vi "testReadNotifierServerStatus_cmd.vi"(8 "error in (no error)":errorcluster) -> (0 "error out":errorcluster)   [LabVIEW 2018]
doc: "Test the readNotifierServerStatus.vi with cmd selection."
uses:
  src/TcpServer/TcpServer.lvclass
  src/TcpServer/TcpServer.lvclass/TcpServer.ctl
  src/TcpServerBase/TcpServerBase.lvclass/TcpServerBase.ctl
  src/TcpServerCmd/TcpServerCmd.lvclass
  home/pcortes/Documents/github/ts_labview_tcp_json/src/TcpServerBase/TcpServerBase.lvclass
  <vilib>/addons/_JKI Toolkits/Caraya/classes/Assert/Assert Equal Type_Variant.vi
  <vilib>/addons/_JKI Toolkits/Caraya/classes/Test/Test.lvclass
  <vilib>/addons/_JKI Toolkits/Caraya/classes/Assert/Assert.lvclass
  src/TcpServerBase/TcpServerBase.lvclass
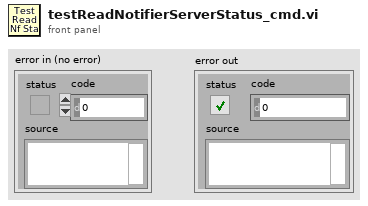
[diagram p1: front panel]
types:
  T1 = cluster{"connectionStatus":bool, "errorSource":string}
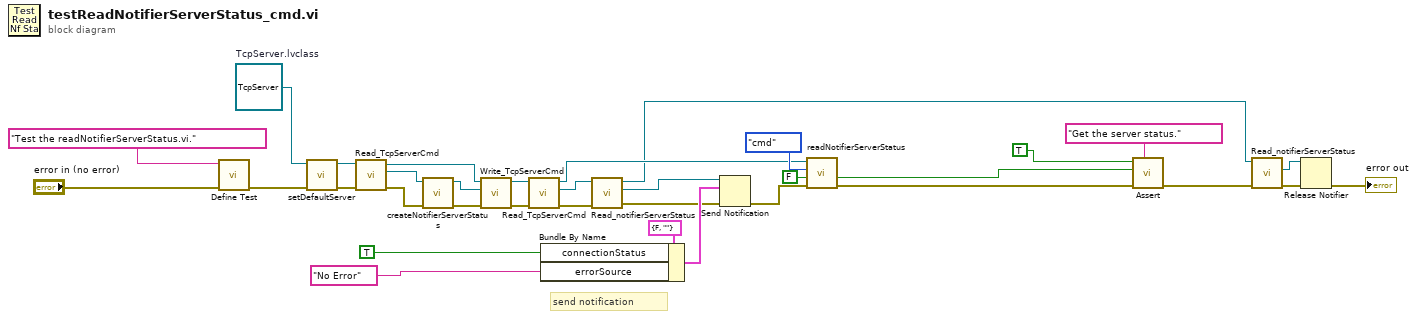
[diagram p0: block diagram]
diagram:
  w29 = refnum<class "TcpServer.lvclass"> refnum  # TcpServer.lvclass
  # "send notification"
  n1 = call <vilib>:"Define Test.vi"("error in (no error)"="error in (no error)", "Label (VI Title)"="Test the readNotifierServerStatus.vi.") -> ("error out"=w28:errorcluster)  [unwired: 9 in]
  n2 = call "setDefaultServer.vi"("error in (no error)"=w28, "TcpServer.lvclass"=w29) -> ("error out"=w27:errorcluster, "tcpServer out"=w26:refnum<class "TcpServer.lvclass">)  [unwired: 8 in]
  n3 = call "Read_TcpServerCmd.vi"("error in (no error)"=w27, "TcpServer in"=w26) -> ("error out"=w12:errorcluster, "TcpServerCmd.lvclass"=w13:refnum<class "TcpServerCmd.lvclass">, "TcpServer out"=w11:refnum<class "TcpServer.lvclass">)  [unwired: 7 in]
  n4 = call "createNotifierServerStatus.vi"("error in (no error)"=w12, "tcpServerBase in"=w13) -> ("error out"=w15:errorcluster, "tcpServerBase out"=w10:refnum<class "TcpServerCmd.lvclass">)  [unwired: 8 in]
  n5 = call "Write_TcpServerCmd.vi"("error in (no error)"=w15, "TcpServerCmd.lvclass"=w10, "TcpServer in"=w11) -> ("error out"=w14:errorcluster, "TcpServer out"=w9:refnum<class "TcpServer.lvclass">)  [unwired: 7 in]
  n6 = call "Read_TcpServerCmd.vi"("error in (no error)"=w14, "TcpServer in"=w9) -> ("error out"=w6:errorcluster, "TcpServerCmd.lvclass"=w7:refnum<class "TcpServerCmd.lvclass">, "TcpServer out"=w8:refnum<class "TcpServer.lvclass">)  [unwired: 7 in]
  n7 = Bundle By Name(cluster=T1 {"connectionStatus"=FALSE, "errorSource"=""} ("notification"), "connectionStatus"=TRUE, "errorSource"="No Error" ("source")) -> (w21:T1)
  n8 = call "Read_notifierServerStatus.vi"("error in (no error)"=w6, "TcpServerBase in"=w7) -> ("error out"=w20:errorcluster, "notifierServerStatus"=w25:refnum<notifier>, "TcpServerBase out"=w1:refnum<class "TcpServerCmd.lvclass">)  [unwired: 7 in]
  n9 = Send Notification(notification=w21, notifier=w25, error in (no error)=w20) -> (error out=w19:errorcluster)  [unwired: 1 out]
  n10 = call "readNotifierServerStatus.vi"("error in (no error)"=w19, "notifierStatusOld"=FALSE ("notification in"), "serverSelection"=enum16{"cmd", "tel"}."cmd", "TcpServer in"=w8) -> ("error out (no error)"=w30:errorcluster, "notifierStatusNew"=w31:bool)  [unwired: 5 in, 1 out]
  n11 = call-poly <vilib>:"Assert.vi"("Label"="Get the server status.", "error in (no error)"=w30, "Y"=w31, "X"=TRUE) -> ("error out"=w3:errorcluster)  [unwired: 7 in]
  n12 = call "Read_notifierServerStatus.vi"("error in (no error)"=w3, "TcpServerBase in"=w1) -> ("error out"=w4:errorcluster, "notifierServerStatus"=w5:refnum<notifier>)  [unwired: 7 in, 1 out]
  n13 = Release Notifier(notifier=w5, error in (no error)=w4) -> (error out=→"error out":errorcluster)  [unwired: 1 in, 2 out]
